vi "Find Virtual Sensor Readings NIARC 2017 Course (SubVI).vi"(7 "Noise":dbl, 8 "Lidar's Maximum Viewing Distance":dbl=5.6, 9 "Lidar Viewing Angle (degrees)":dbl=240.0, 10 "Number of Lidar Measurements":dbl=683.0, 11 "Position":cluster{"X":dbl, "Y":dbl, "Angle":dbl}) -> (0 "Polar Plot":picture, 1 "Angle":dbl[](array[numeric]), 2 "Magnitude":dbl[](array[numeric]))   [LabVIEW 2016]
uses:
  <vilib>/ptbypt/NI_PtbyPt.lvlib
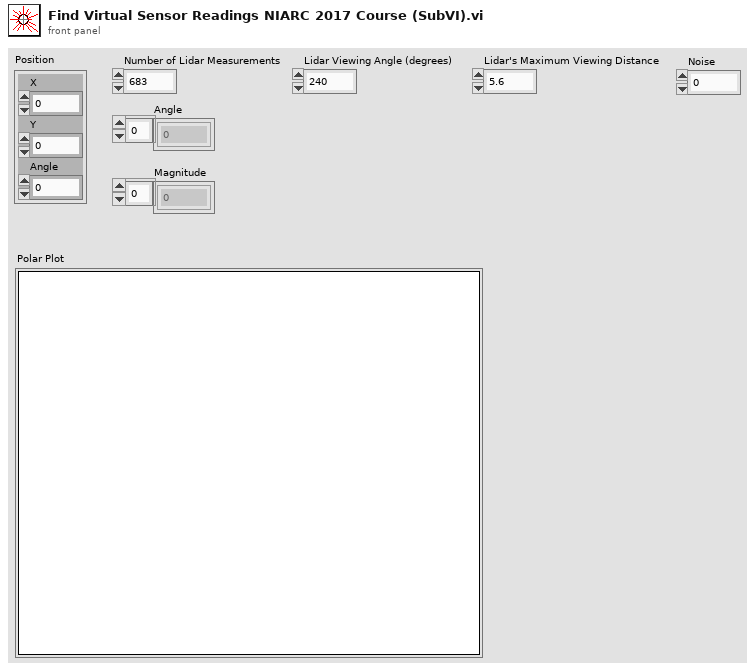
[diagram p1: front panel]
types:
  T1 = typedef "LVBoundsTypeDef.ctl" = cluster{"Width":u32, "Height":u32}
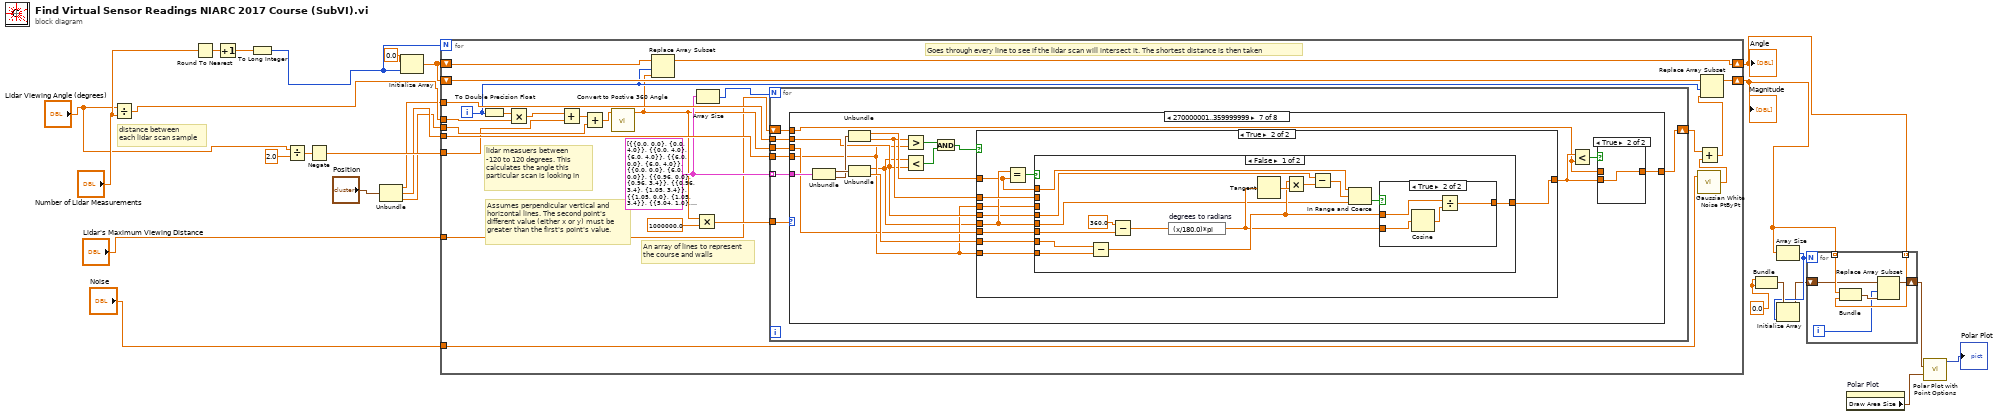
[diagram p0: block diagram]
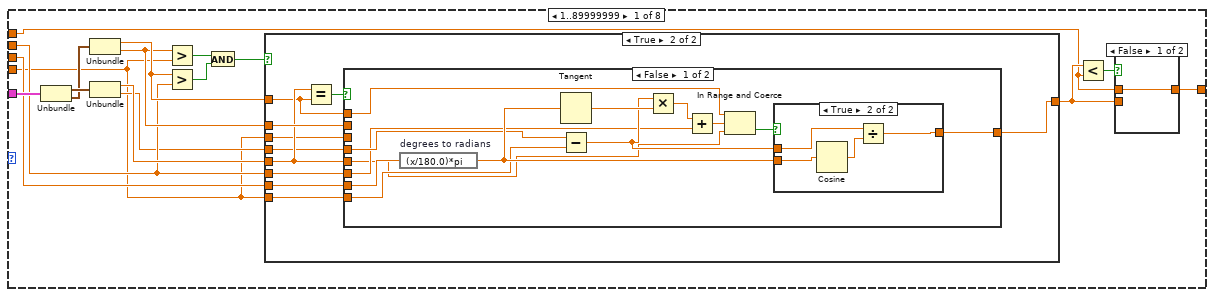
[diagram p2: hidden frame]
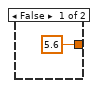
[diagram p4: hidden frame]
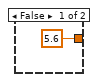
[diagram p5: hidden frame]
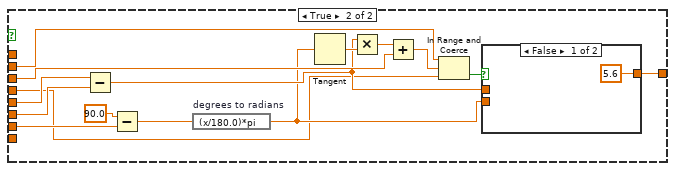
[diagram p6: hidden frame]
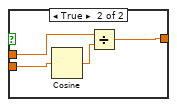
[diagram p7: hidden frame]
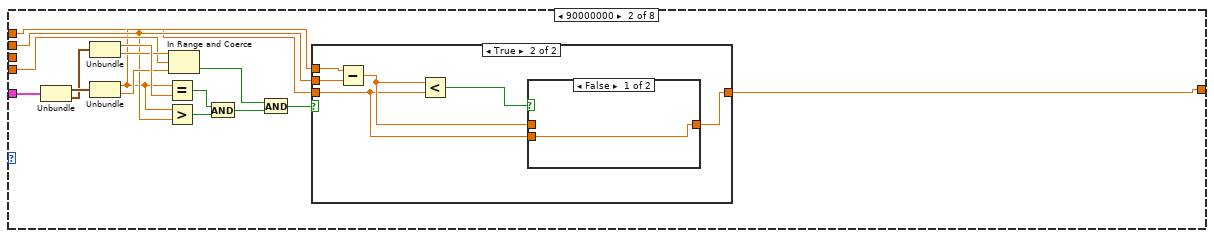
[diagram p8: hidden frame]
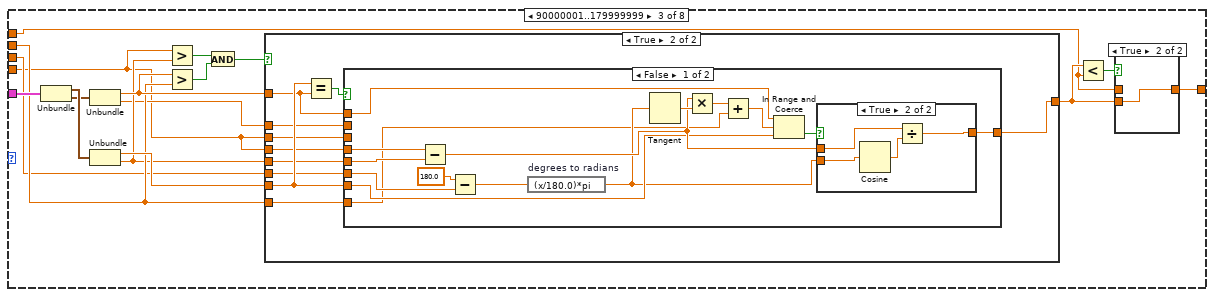
[diagram p11: hidden frame]
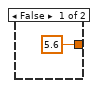
[diagram p13: hidden frame]
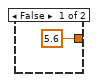
[diagram p14: hidden frame]
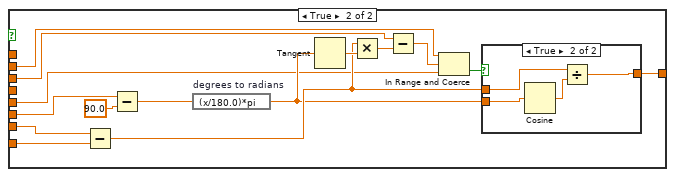
[diagram p15: hidden frame]
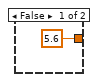
[diagram p16: hidden frame]
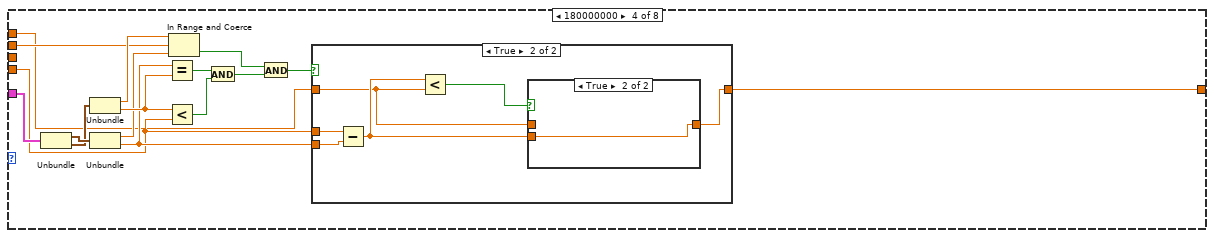
[diagram p17: hidden frame]
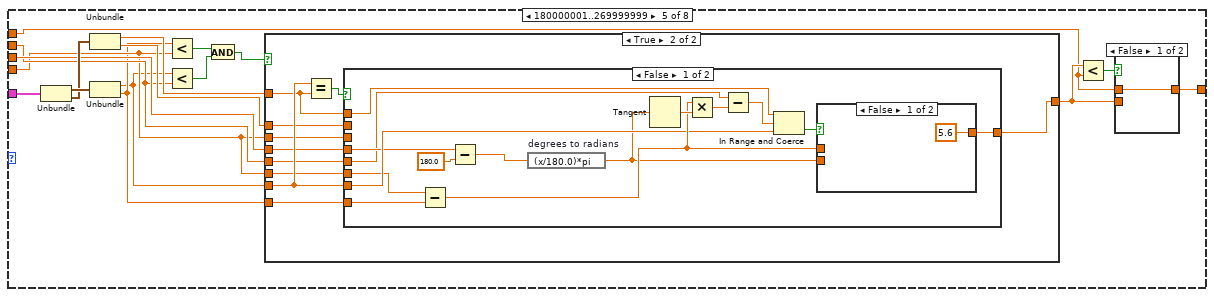
[diagram p20: hidden frame]
diagram:
  w5 = 0.0
  # "distance between\neach lidar scan sample"
  n1 = Divide(x="Lidar Viewing Angle (degrees)", y="Number of Lidar Measurements") -> (x/y=w23:dbl)
  n2 = Round To Nearest(number="Number of Lidar Measurements") -> (nearest integer value=w26:dbl)
  n3 = Increment(x=w26) -> (x+1=w25:dbl)
  n4 = To Long Integer(number=w25) -> (32bit integer=w24:i32)
  n5 = Divide(x="Lidar Viewing Angle (degrees)", y=2.0) -> (x/y=w20:dbl)
  n6 = Negate(x=w20) -> (-x=w17:dbl)
  n7 = Unbundle("Position") -> ("X"=w13:dbl, "Y"=w12:dbl, "Angle"=w11:dbl)
  n8 = Initialize Array(0.0 ("element"), w24) -> (w15:dbl[])
  n9 = for {
    N: w24 -> [_]
    tunnel: w11 -> [w44]
    tunnel: w13 -> [w49]
    tunnel: w12 -> [w48]
    tunnel: w23 -> [w47]
    shift-right: [w41] -> w8
    shift-left: w15 -> [w42]
    shift-right: [w33] -> w7
    shift-left: w15 -> [w35]
    tunnel: "Lidar's Maximum Viewing Distance" -> [w32]
    tunnel: w17 -> [w31]
    tunnel: "Noise" -> [w27]
    i -> [w36]
    w40 = cluster{cluster{dbl, dbl}, cluster{dbl, dbl}}[] [{{0.0, 0.0}, {0.0, 4.0}}, {{0.0, 4.0}, {6.0, 4.0}}, {{6.0, 0.0}, {6.0, 4.0}}, {{0.0, 0.0}, {6.0, 0.0}}, {{0.96, 0.0}, {0.96, 3.4}}, {{0.96, 3.4}, {1.05, 3.4}}, {{1.05, 0.0}, {1.05, 3.4}}, {{5.04, 1.0}, {5.04, 3.4}}, {{4.95, 1.0}, {5.04, 1.0}}, {{4.95, 1.0}, {4.95, 3.4}}, {{4.95, 3.4}, {5.04, 3.4}}, {{1.65, 1.0}, {4.35, 1.0}}, {{0.0, 0.0}, {0.0, 0.0}}]
    # "Assumes perpendicular vertical and\nhorizontal lines. The second point's\ndifferent value (either x or y) must be\ngreater than the first's point's value."
    # "Goes through every line to see if the lidar scan will intersect it. The shortest distance is then taken"
    # "An array of lines to represent\nthe course and walls"
    # "lidar measuers between\n-120 to 120 degrees. This\ncalculates the angle this \nparticular scan is looking in"
    n10 = To Double Precision Float(number=w36) -> (double precision float=w46:dbl)
    n11 = Multiply(x=w46, y=w47) -> (x*y=w45:dbl)
    n12 = Add(x=w45, y=w31) -> (x+y=w43:dbl)
    n13 = Add(x=w43, y=w44) -> (x+y=w37:dbl)
    n14 = call "Convert to Postive 360 Angle.vi"("Angle in"=w37) -> ("Angle out"=w34:dbl)  [unwired: 10 in]
    n15 = Replace Array Subset(array=w35, new element=w34, index=w36) -> (w33:dbl[])
    n16 = Multiply(x=w34, y=1000000.0) -> (x*y=w38:dbl)
    n17 = Array Size(array=w40) -> (size(s)=w50:i32)
    n18 = for {
      N: w50 -> [_]
      tunnel: w40 -> [w57] mode=indexing
      tunnel: w48 -> [w56]
      tunnel: w49 -> [w55]
      shift-right: [w53] -> w29
      shift-left: w32 -> [w54]
      tunnel: w34 -> [w52]
      tunnel: w38 -> [w51]
      n19 = case shown="270000001..359999999" w51 {
        tunnel: w57 -> [w72 w134 w159 w225 w253 w320 w347 w426]
        tunnel: w56 -> [w58 w130 w151 w224 w249 w317 w343 w413]
        tunnel: w55 -> [w65 w129 w157 w223 w251 w316 w344 w420]
        tunnel: w54 -> [w60 w127 w152 w222 w250 w318 w345 w412]
        tunnel: [w62 w126 w153 w221 w246 w319 w342 w411] -> w53
        tunnel: w52 -> [w64 _ w156 _ w252 _ w346 _]
        frame 1..89999999 {
          n20 = Unbundle(w72) -> (w74:cluster{dbl, dbl}, w73:cluster{dbl, dbl})
          n21 = Unbundle(w73) -> (w67:dbl, w66:dbl)
          n22 = Unbundle(w74) -> (w68:dbl, w59:dbl)
          n23 = Greater?(x=w66, y=w58) -> (0:w71:bool)
          n24 = Greater?(x=w67, y=w65) -> (0:w70:bool)
          n25 = And(x=w71, y=w70) -> (x .and. y?=w69:bool)
          n26 = case shown="True" w69 {
            tunnel: [5.6 w81] -> w61
            tunnel: w68 -> [_ w85]
            tunnel: w67 -> [_ w78]
            tunnel: w66 -> [_ w86]
            tunnel: w65 -> [_ w84]
            tunnel: w64 -> [_ w83]
            tunnel: w58 -> [_ w82]
            tunnel: w59 -> [_ w80]
            tunnel: w58 -> [_ w79]
            frame False {
            }
            frame True {
              n27 = Equal?(x=w85, y=w78) -> (x = y?=w87:bool)
              n28 = case shown="False" w87 {
                tunnel: w86 -> [_ w109]
                tunnel: w85 -> [w88 w120]
                tunnel: w84 -> [w93 w119]
                tunnel: w83 -> [w94 w118]
                tunnel: w82 -> [_ w113]
                tunnel: [w92 w110] -> w81
                tunnel: w80 -> [w96 w108]
                tunnel: w79 -> [w95 _]
                tunnel: w78 -> [w91 _]
                frame False {
                  n29 = expression code="(x/180.0)*pi" "degrees to radians"(w94) -> (w97:dbl)
                  n30 = Tangent(1:w97) -> (0:w100:dbl)
                  n31 = Subtract(x=w96, y=w95) -> (x-y=w98:dbl)
                  n32 = Multiply(x=w98, y=w100) -> (x*y=w99:dbl)
                  n33 = Add(x=w99, y=w93) -> (x+y=w90:dbl)
                  n34 = In Range and Coerce(upper limit=w91, x=w90, lower limit=w88) -> (In Range?=w89:bool)  [unwired: 1 out]
                  n35 = case shown="True" w89 {
                    tunnel: w98 -> [_ w105]
                    tunnel: w97 -> [_ w103]
                    tunnel: [5.6 w102] -> w92
                    frame False {
                    }
                    frame True {
                      n36 = Cosine(x=w103) -> (cos(x)=w104:dbl)
                      n37 = Divide(x=w105, y=w104) -> (x/y=w102:dbl)
                    }
                  }
                }
                frame True {
                  n38 = Subtract(x=w120, y=w119) -> (x-y=w112:dbl)
                  n39 = Subtract(x=90.0, y=w118) -> (x-y=w116:dbl)
                  n40 = expression code="(x/180.0)*pi" "degrees to radians"(w116) -> (w111:dbl)
                  n41 = Tangent(1:w111) -> (0:w115:dbl)
                  n42 = Multiply(x=w112, y=w115) -> (x*y=w114:dbl)
                  n43 = Add(x=w114, y=w113) -> (x+y=w107:dbl)
                  n44 = In Range and Coerce(upper limit=w109, x=w107, lower limit=w108) -> (In Range?=w106:bool)  [unwired: 1 out]
                  n45 = case shown="False" w106 {
                    tunnel: w112 -> [_ w125]
                    tunnel: w111 -> [_ w123]
                    tunnel: [5.6 w122] -> w110
                    frame False {
                    }
                    frame True {
                      n46 = Cosine(x=w123) -> (cos(x)=w124:dbl)
                      n47 = Divide(x=w125, y=w124) -> (x/y=w122:dbl)
                    }
                  }
                }
              }
            }
          }
          n48 = Less?(x=w61, y=w60) -> (x < y?=w63:bool)
          n49 = case shown="False" w63 {
            tunnel: [w75 w76] -> w62
            tunnel: w61 -> [_ w76]
            tunnel: w60 -> [w75 _]
            frame False {
            }
            frame True {
            }
          }
        }
        frame 90000000 {
          n50 = Unbundle(w134) -> (w141:cluster{dbl, dbl}, w140:cluster{dbl, dbl})
          n51 = Unbundle(w140) -> (w133:dbl, w131:dbl)
          n52 = Unbundle(w141) -> (w128:dbl, w132:dbl)
          n53 = Equal?(x=w128, y=w133) -> (x = y?=w138:bool)
          n54 = Greater?(x=w128, y=w129) -> (0:w139:bool)
          n55 = In Range and Coerce(upper limit=w131, x=w130, lower limit=w132) -> (In Range?=w136:bool)  [unwired: 1 out]
          n56 = And(x=w138, y=w139) -> (x .and. y?=w137:bool)
          n57 = And(x=w136, y=w137) -> (x .and. y?=w135:bool)
          n58 = case shown="True" w135 {
            tunnel: [w142 w147] -> w126
            tunnel: w129 -> [_ w145]
            tunnel: w128 -> [_ w144]
            tunnel: w127 -> [w142 w143]
            frame False {
            }
            frame True {
              n59 = Subtract(x=w144, y=w145) -> (x-y=w146:dbl)
              n60 = Less?(x=w146, y=w143) -> (x < y?=w148:bool)
              n61 = case shown="False" w148 {
                tunnel: [w149 w150] -> w147
                tunnel: w146 -> [_ w150]
                tunnel: w143 -> [w149 _]
                frame False {
                }
                frame True {
                }
              }
            }
          }
        }
        frame 90000001..179999999 {
          n62 = Unbundle(w159) -> (w167:cluster{dbl, dbl}, w166:cluster{dbl, dbl})
          n63 = Unbundle(w166) -> (w158:dbl, w154:dbl)
          n64 = Unbundle(w167) -> (w162:dbl, w155:dbl)
          n65 = Greater?(x=w151, y=w155) -> (0:w165:bool)
          n66 = Greater?(x=w158, y=w157) -> (0:w164:bool)
          n67 = And(x=w165, y=w164) -> (x .and. y?=w163:bool)
          n68 = case shown="True" w163 {
            tunnel: [5.6 w178] -> w160
            tunnel: w162 -> [_ w179]
            tunnel: w158 -> [_ w176]
            tunnel: w155 -> [_ w177]
            tunnel: w157 -> [_ w175]
            tunnel: w156 -> [_ w174]
            tunnel: w151 -> [_ w173]
            tunnel: w154 -> [_ w172]
            tunnel: w151 -> [_ w171]
            frame False {
            }
            frame True {
              n69 = Equal?(x=w179, y=w176) -> (x = y?=w180:bool)
              n70 = case shown="False" w180 {
                tunnel: w179 -> [w188 w215]
                tunnel: [w192 w210] -> w178
                tunnel: w177 -> [w187 w209]
                tunnel: w176 -> [w191 _]
                tunnel: w175 -> [w181 w207]
                tunnel: w174 -> [w183 w205]
                tunnel: w173 -> [_ w202]
                tunnel: w172 -> [_ w201]
                tunnel: w171 -> [w186 _]
                frame False {
                  n71 = Subtract(x=w186, y=w187) -> (x-y=w193:dbl)
                  n72 = Subtract(x=180.0, y=w183) -> (x-y=w185:dbl)
                  n73 = expression code="(x/180.0)*pi" "degrees to radians"(w185) -> (w182:dbl)
                  n74 = Tangent(1:w182) -> (0:w195:dbl)
                  n75 = Multiply(x=w193, y=w195) -> (x*y=w194:dbl)
                  n76 = Add(x=w194, y=w181) -> (x+y=w190:dbl)
                  n77 = In Range and Coerce(upper limit=w191, x=w190, lower limit=w188) -> (In Range?=w189:bool)  [unwired: 1 out]
                  n78 = case shown="True" w189 {
                    tunnel: w193 -> [_ w200]
                    tunnel: w182 -> [_ w198]
                    tunnel: [5.6 w197] -> w192
                    frame False {
                    }
                    frame True {
                      n79 = Cosine(x=w198) -> (cos(x)=w199:dbl)
                      n80 = Divide(x=w200, y=w199) -> (x/y=w197:dbl)
                    }
                  }
                }
                frame True {
                  n81 = Subtract(x=w215, y=w207) -> (x-y=w212:dbl)
                  n82 = Subtract(x=w205, y=90.0 ("x")) -> (x-y=w214:dbl)
                  n83 = expression code="(x/180.0)*pi" "degrees to radians"(w214) -> (w211:dbl)
                  n84 = Tangent(1:w211) -> (0:w213:dbl)
                  n85 = Multiply(x=w212, y=w213) -> (x*y=w203:dbl)
                  n86 = Subtract(x=w202, y=w203) -> (x-y=w204:dbl)
                  n87 = In Range and Coerce(upper limit=w201, x=w204, lower limit=w209) -> (In Range?=w208:bool)  [unwired: 1 out]
                  n88 = case shown="True" w208 {
                    tunnel: w212 -> [_ w220]
                    tunnel: w211 -> [_ w218]
                    tunnel: [5.6 w217] -> w210
                    frame False {
                    }
                    frame True {
                      n89 = Cosine(x=w218) -> (cos(x)=w219:dbl)
                      n90 = Divide(x=w220, y=w219) -> (x/y=w217:dbl)
                    }
                  }
                }
              }
            }
          }
          n91 = Less?(x=w160, y=w152) -> (x < y?=w161:bool)
          n92 = case shown="True" w161 {
            tunnel: [w168 w169] -> w153
            tunnel: w160 -> [_ w169]
            tunnel: w152 -> [w168 _]
            frame False {
            }
            frame True {
            }
          }
        }
        frame 180000000 {
          n93 = Unbundle(w225) -> (w236:cluster{dbl, dbl}, w235:cluster{dbl, dbl})
          n94 = Unbundle(w235) -> (w230:dbl, w234:dbl)
          n95 = Unbundle(w236) -> (w231:dbl, w226:dbl)
          n96 = Equal?(x=w226, y=w234) -> (x = y?=w232:bool)
          n97 = Less?(x=w234, y=w224) -> (x < y?=w233:bool)
          n98 = In Range and Coerce(upper limit=w230, x=w223, lower limit=w231) -> (In Range?=w228:bool)  [unwired: 1 out]
          n99 = And(x=w232, y=w233) -> (x .and. y?=w229:bool)
          n100 = And(x=w228, y=w229) -> (x .and. y?=w227:bool)
          n101 = case shown="True" w227 {
            tunnel: w226 -> [_ w238]
            tunnel: w224 -> [_ w239]
            tunnel: w222 -> [w237 w240]
            tunnel: [w237 w242] -> w221
            frame False {
            }
            frame True {
              n102 = Subtract(x=w239, y=w238) -> (x-y=w241:dbl)
              n103 = Less?(x=w241, y=w240) -> (x < y?=w243:bool)
              n104 = case shown="True" w243 {
                tunnel: [w244 w245] -> w242
                tunnel: w241 -> [_ w245]
                tunnel: w240 -> [w244 _]
                frame False {
                }
                frame True {
                }
              }
            }
          }
        }
        frame 180000001..269999999 {
          n105 = Unbundle(w253) -> (w262:cluster{dbl, dbl}, w261:cluster{dbl, dbl})
          n106 = Unbundle(w261) -> (w255:dbl, w254:dbl)
          n107 = Unbundle(w262) -> (w247:dbl, w248:dbl)
          n108 = Less?(x=w248, y=w249) -> (x < y?=w260:bool)
          n109 = Less?(x=w247, y=w251) -> (x < y?=w259:bool)
          n110 = And(x=w260, y=w259) -> (x .and. y?=w258:bool)
          n111 = case shown="True" w258 {
            tunnel: [5.6 w273] -> w256
            tunnel: w247 -> [_ w274]
            tunnel: w255 -> [_ w271]
            tunnel: w248 -> [_ w272]
            tunnel: w251 -> [_ w270]
            tunnel: w252 -> [_ w269]
            tunnel: w249 -> [_ w268]
            tunnel: w254 -> [_ w267]
            tunnel: w249 -> [_ w266]
            frame False {
            }
            frame True {
              n112 = Equal?(x=w274, y=w271) -> (x = y?=w275:bool)
              n113 = case shown="False" w275 {
                tunnel: w274 -> [w284 w297]
                tunnel: [w288 w306] -> w273
                tunnel: w272 -> [w283 w305]
                tunnel: w271 -> [w287 _]
                tunnel: w270 -> [w276 w296]
                tunnel: w269 -> [w279 w298]
                tunnel: w268 -> [_ w301]
                tunnel: w267 -> [_ w300]
                tunnel: w266 -> [w282 _]
                frame False {
                  n114 = Subtract(x=w282, y=w283) -> (x-y=w289:dbl)
                  n115 = Subtract(x=w279, y=180.0 ("x")) -> (x-y=w278:dbl)
                  n116 = expression code="(x/180.0)*pi" "degrees to radians"(w278) -> (w281:dbl)
                  n117 = Tangent(1:w281) -> (0:w290:dbl)
                  n118 = Multiply(x=w289, y=w290) -> (x*y=w277:dbl)
                  n119 = Subtract(x=w276, y=w277) -> (x-y=w286:dbl)
                  n120 = In Range and Coerce(upper limit=w287, x=w286, lower limit=w284) -> (In Range?=w285:bool)  [unwired: 1 out]
                  n121 = case shown="False" w285 {
                    tunnel: w289 -> [_ w295]
                    tunnel: w281 -> [_ w293]
                    tunnel: [5.6 w292] -> w288
                    frame False {
                    }
                    frame True {
                      n122 = Cosine(x=w293) -> (cos(x)=w294:dbl)
                      n123 = Divide(x=w295, y=w294) -> (x/y=w292:dbl)
                    }
                  }
                }
                frame True {
                  n124 = Subtract(x=w296, y=w297) -> (x-y=w308:dbl)
                  n125 = Subtract(x=270.0, y=w298) -> (x-y=w310:dbl)
                  n126 = expression code="(x/180.0)*pi" "degrees to radians"(w310) -> (w307:dbl)
                  n127 = Tangent(1:w307) -> (0:w309:dbl)
                  n128 = Multiply(x=w308, y=w309) -> (x*y=w302:dbl)
                  n129 = Subtract(x=w301, y=w302) -> (x-y=w303:dbl)
                  n130 = In Range and Coerce(upper limit=w300, x=w303, lower limit=w305) -> (In Range?=w304:bool)  [unwired: 1 out]
                  n131 = case shown="True" w304 {
                    tunnel: w308 -> [_ w315]
                    tunnel: w307 -> [_ w313]
                    tunnel: [5.6 w312] -> w306
                    frame False {
                    }
                    frame True {
                      n132 = Cosine(x=w313) -> (cos(x)=w314:dbl)
                      n133 = Divide(x=w315, y=w314) -> (x/y=w312:dbl)
                    }
                  }
                }
              }
            }
          }
          n134 = Less?(x=w256, y=w250) -> (x < y?=w257:bool)
          n135 = case shown="False" w257 {
            tunnel: [w263 w264] -> w246
            tunnel: w256 -> [_ w264]
            tunnel: w250 -> [w263 _]
            frame False {
            }
            frame True {
            }
          }
        }
        frame 270000000 {
          n136 = Unbundle(w320) -> (w331:cluster{dbl, dbl}, w330:cluster{dbl, dbl})
          n137 = Unbundle(w330) -> (w324:dbl, w322:dbl)
          n138 = Unbundle(w331) -> (w321:dbl, w323:dbl)
          n139 = Equal?(x=w321, y=w324) -> (x = y?=w328:bool)
          n140 = Less?(x=w321, y=w316) -> (x < y?=w329:bool)
          n141 = In Range and Coerce(upper limit=w322, x=w317, lower limit=w323) -> (In Range?=w326:bool)  [unwired: 1 out]
          n142 = And(x=w328, y=w329) -> (x .and. y?=w327:bool)
          n143 = And(x=w326, y=w327) -> (x .and. y?=w325:bool)
          n144 = case shown="True" w325 {
            tunnel: [w332 w337] -> w319
            tunnel: w316 -> [_ w335]
            tunnel: w321 -> [_ w334]
            tunnel: w318 -> [w332 w333]
            frame False {
            }
            frame True {
              n145 = Subtract(x=w335, y=w334) -> (x-y=w336:dbl)
              n146 = Less?(x=w336, y=w333) -> (x < y?=w338:bool)
              n147 = case shown="False" w338 {
                tunnel: [w339 w340] -> w337
                tunnel: w336 -> [_ w340]
                tunnel: w333 -> [w339 _]
                frame False {
                }
                frame True {
                }
              }
            }
          }
        }
        frame 270000001..359999999 {
          n148 = Unbundle(w347) -> (w357:cluster{dbl, dbl}, w356:cluster{dbl, dbl})
          n149 = Unbundle(w356) -> (w352:dbl, w351:dbl)
          n150 = Unbundle(w357) -> (w341:dbl, w348:dbl)
          n151 = Greater?(x=w351, y=w343) -> (0:w355:bool)
          n152 = Less?(x=w341, y=w344) -> (x < y?=w354:bool)
          n153 = And(x=w355, y=w354) -> (x .and. y?=w353:bool)
          n154 = case shown="True" w353 {
            tunnel: [5.6 w364] -> w349
            tunnel: w341 -> [_ w368]
            tunnel: w352 -> [_ w361]
            tunnel: w351 -> [_ w369]
            tunnel: w344 -> [_ w367]
            tunnel: w346 -> [_ w366]
            tunnel: w343 -> [_ w365]
            tunnel: w348 -> [_ w363]
            tunnel: w343 -> [_ w362]
            frame False {
            }
            frame True {
              n155 = Equal?(x=w368, y=w361) -> (x = y?=w370:bool)
              n156 = case shown="False" w370 {
                tunnel: w369 -> [_ w398]
                tunnel: w368 -> [w376 w394]
                tunnel: w367 -> [w373 w393]
                tunnel: w366 -> [w371 w391]
                tunnel: w365 -> [_ w402]
                tunnel: [w380 w399] -> w364
                tunnel: w363 -> [w382 w397]
                tunnel: w362 -> [w381 _]
                tunnel: w361 -> [w379 _]
                frame False {
                  n157 = Subtract(x=w382, y=w381) -> (x-y=w384:dbl)
                  n158 = Subtract(x=360.0 ("y"), y=w371) -> (x-y=w375:dbl)
                  n159 = expression code="(x/180.0)*pi" "degrees to radians"(w375) -> (w383:dbl)
                  n160 = Tangent(1:w383) -> (0:w385:dbl)
                  n161 = Multiply(x=w384, y=w385) -> (x*y=w374:dbl)
                  n162 = Subtract(x=w373, y=w374) -> (x-y=w378:dbl)
                  n163 = In Range and Coerce(upper limit=w379, x=w378, lower limit=w376) -> (In Range?=w377:bool)  [unwired: 1 out]
                  n164 = case shown="True" w377 {
                    tunnel: w384 -> [_ w390]
                    tunnel: w383 -> [_ w388]
                    tunnel: [5.6 w387] -> w380
                    frame False {
                    }
                    frame True {
                      n165 = Cosine(x=w388) -> (cos(x)=w389:dbl)
                      n166 = Divide(x=w390, y=w389) -> (x/y=w387:dbl)
                    }
                  }
                }
                frame True {
                  n167 = Subtract(x=w393, y=w394) -> (x-y=w401:dbl)
                  n168 = Subtract(x=w391, y=270.0 ("x")) -> (x-y=w405:dbl)
                  n169 = expression code="(x/180.0)*pi" "degrees to radians"(w405) -> (w400:dbl)
                  n170 = Tangent(1:w400) -> (0:w404:dbl)
                  n171 = Multiply(x=w401, y=w404) -> (x*y=w403:dbl)
                  n172 = Add(x=w403, y=w402) -> (x+y=w396:dbl)
                  n173 = In Range and Coerce(upper limit=w398, x=w396, lower limit=w397) -> (In Range?=w395:bool)  [unwired: 1 out]
                  n174 = case shown="True" w395 {
                    tunnel: w401 -> [_ w410]
                    tunnel: w400 -> [_ w408]
                    tunnel: [5.6 w407] -> w399
                    frame False {
                    }
                    frame True {
                      n175 = Cosine(x=w408) -> (cos(x)=w409:dbl)
                      n176 = Divide(x=w410, y=w409) -> (x/y=w407:dbl)
                    }
                  }
                }
              }
            }
          }
          n177 = Less?(x=w349, y=w345) -> (x < y?=w350:bool)
          n178 = case shown="True" w350 {
            tunnel: [w358 w359] -> w342
            tunnel: w349 -> [_ w359]
            tunnel: w345 -> [w358 _]
            frame False {
            }
            frame True {
            }
          }
        }
        frame 0, Default {
          n179 = Unbundle(w426) -> (w425:cluster{dbl, dbl}, w424:cluster{dbl, dbl})
          n180 = Unbundle(w424) -> (w418:dbl, w423:dbl)
          n181 = Unbundle(w425) -> (w419:dbl, w414:dbl)
          n182 = Equal?(x=w414, y=w423) -> (x = y?=w421:bool)
          n183 = Greater?(x=w423, y=w413) -> (0:w422:bool)
          n184 = In Range and Coerce(upper limit=w418, x=w420, lower limit=w419) -> (In Range?=w416:bool)  [unwired: 1 out]
          n185 = And(x=w421, y=w422) -> (x .and. y?=w417:bool)
          n186 = And(x=w416, y=w417) -> (x .and. y?=w415:bool)
          n187 = case shown="True" w415 {
            tunnel: w414 -> [_ w433]
            tunnel: w413 -> [_ w432]
            tunnel: w412 -> [w427 w428]
            tunnel: [w427 w430] -> w411
            frame False {
            }
            frame True {
              n188 = Subtract(x=w433, y=w432) -> (x-y=w429:dbl)
              n189 = Less?(x=w429, y=w428) -> (x < y?=w431:bool)
              n190 = case shown="False" w431 {
                tunnel: [w434 w435] -> w430
                tunnel: w429 -> [_ w435]
                tunnel: w428 -> [w434 _]
                frame False {
                }
                frame True {
                }
              }
            }
          }
        }
      }
    }
    n191 = call <vilib>:"Gaussian White Noise PtByPt.vi"("standard deviation"=w27) -> ("Gaussian white noise"=w30:dbl)  [unwired: 2 in]
    n192 = Add(x=w29, y=w30) -> (x+y=w28:dbl)
    n193 = Replace Array Subset(array=w42, new element=w28, index=w36) -> (w41:dbl[])
  }
  "Angle" <- w7
  "Magnitude" <- w8
  n194 = Bundle(w5, w5) -> (w6:cluster{dbl, dbl})  [unwired: 1 in]
  n195 = Array Size(array=w8) -> (size(s)=w4:i32)
  n196 = Initialize Array(w6, w4) -> (w3:cluster{dbl, dbl}[])
  n197 = for {
    N: w4 -> [_]
    tunnel: w8 -> [w441] mode=indexing
    tunnel: w7 -> [w440] mode=indexing
    shift-right: [w436] -> w2
    shift-left: w3 -> [w437]
    i -> [w438]
    n198 = Bundle("element"=w441, "element"=w440) -> (w439:cluster{"element":dbl, "element":dbl})  [unwired: 1 in]
    n199 = Replace Array Subset(array=w437, new element=w439, index=w438) -> (w436:cluster{dbl, dbl}[])
  }
  n200 = property on="Polar Plot" class="Pict"() -> ("Draw Area Size"=w9:T1)  [unwired: 2 in, 2 out]
  n201 = call <vilib>:"Polar Plot with Point Options.vi"("data array [mag, phase (deg)]"=w2, "dimensions (w,h)"=w9) -> ("new picture"=→"Polar Plot":picture)  [unwired: 13 in]
